vi "RPushX.vi"(0 "reference in":refnum<class "Redis.lvclass">, 1 "Key":string, 7 "Values":string[](array[string]), 11 "Error In":errorcluster) -> (4 "reference out":refnum<class "Redis.lvclass">, 8 "Data":T1, 15 "Error Out":errorcluster)   [LabVIEW 2020, in "Redis.lvclass"]
doc: "<b>RPUSHX</b>\n\nInserts specified values at the tail of the list stored at key, only if key already exists and holds a list. In contrary to RPUSH, no operation will be performed when key does not yet exist."
uses:
  Redis.lvclass
  ReplyDataTypeEnum.ctl
  RedisDataType.ctl
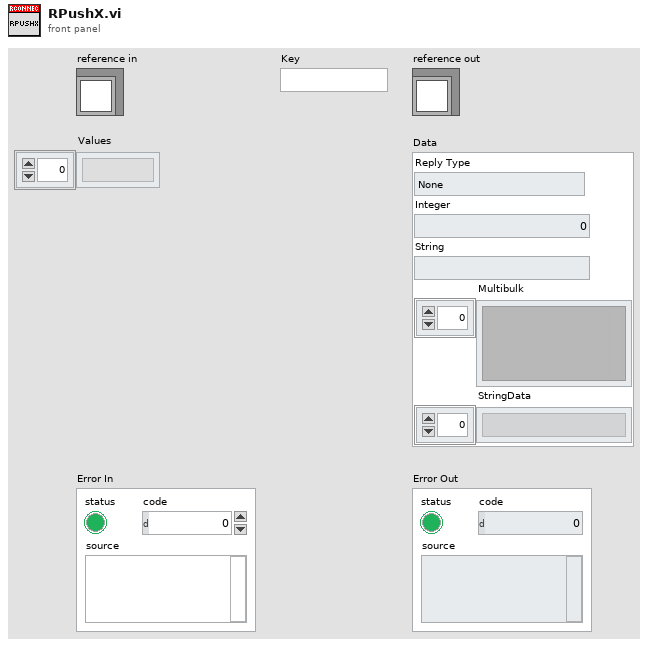
[diagram p1: front panel]
types:
  T1 = typedef "Redis.lvclass/RedisDataType.ctl" = cluster{"Reply Type":T2, "Integer":i64, "String":string, "Multibulk":variant[], "StringData":string[]}
  T2 = typedef "Redis.lvclass/ReplyDataTypeEnum.ctl" = enum16{"None", "Error", "Status", "Nil", "Integer", "String", "Multibulk"}
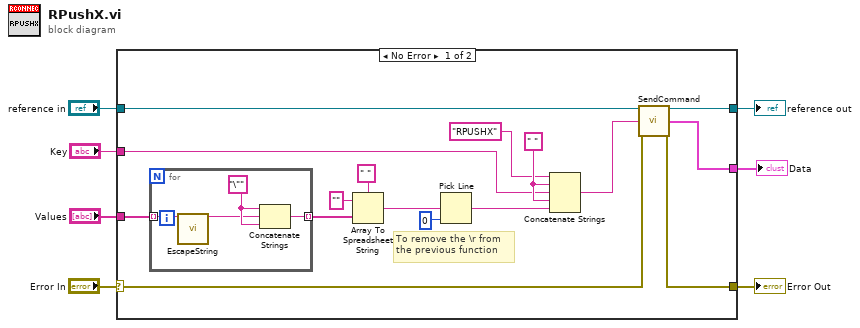
[diagram p0: block diagram]
diagram:
  n1 = case shown="No Error" "Error In" {
    selector: "Error In" -> [w21 w29]
    tunnel: [w20 w29] -> w6
    tunnel: [w23 w28] -> w4
    tunnel: "reference in" -> [w22 w28]
    tunnel: [w19 _] -> w3
    tunnel: "Key" -> [w10 _]
    tunnel: "Values" -> [w9 _]
    frame No Error {
      w13 = " "
      # "To remove the \\r from\nthe previous function"
      n2 = for {
        tunnel: w9 -> [w24] mode=indexing
        tunnel: [w27] -> w12 mode=indexing
        w26 = "\""
        n3 = call "EscapeString.vi"("String"=w24) -> ("Escaped String"=w25:string)  [unwired: 13 in, 1 out]
        n4 = Concatenate Strings(w26, w25, w26) -> (w27:string)
      }
      n5 = Array To Spreadsheet String(delimiter (Tab)=" ", array=w12, 3:"" ("format string")) -> (spreadsheet string=w15:string)
      n6 = Pick Line(multi-line string=w15, line index=0) -> (output string=w16:string)  [unwired: 1 in]
      n7 = Concatenate Strings("RPUSHX", w13, w10, w13, w16) -> (w8:string)
      n8 = call "SendCommand.vi"("reference in"=w22, "Command"=w8, "Error In"=w21) -> ("reference out"=w23:refnum<class "Redis.lvclass">, "Data"=w19:T1, "Error Out"=w20:errorcluster)  [unwired: 10 in]
    }
    frame Error {
    }
  }
  "Error Out" <- w6
  "reference out" <- w4
  "Data" <- w3
